vi "check running.vi"() -> ()   [LabVIEW 2025]
panel:
  out "running":u8
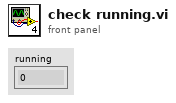
[diagram p1: front panel]
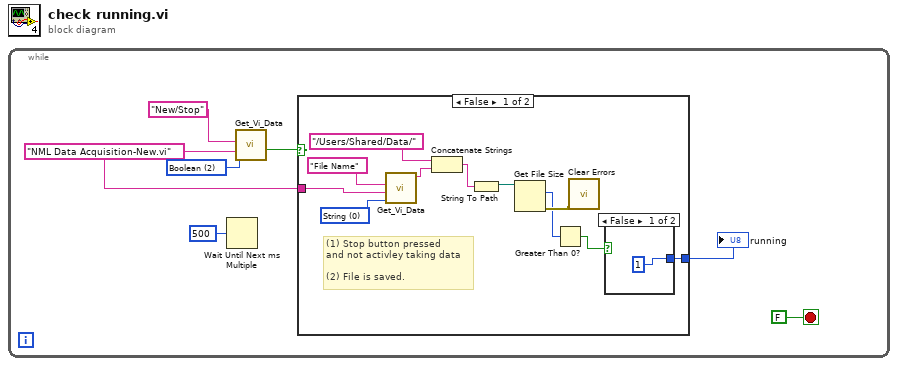
[diagram p0: block diagram]
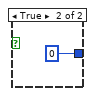
[diagram p2: hidden frame]
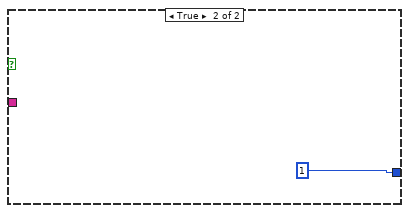
[diagram p3: hidden frame]
diagram:
  n1 = while {
    stop <- FALSE stop-if-true
    w6 = u16 2 items=["String", "Double", "Boolean", "Variant"] ("Data Type")
    w2 = "NML Data Acquisition-New.vi" ("VI name")
    n2 = Wait Until Next ms Multiple(millisecond multiple=u32 500) -> ()  [unwired: 1 out]
    n3 = call "Get_Vi_Data.vi"("Data Type"=w6, "VI name"=w2, "Control Name"="New/Stop") -> ("Boolean"=w5:bool)  [unwired: 4 in, 4 out]
    n4 = case shown="False" w5 {
      tunnel: w2 -> [w18 _]
      tunnel: [w12 u8 1 ("running")] -> w1
      frame False {
        w16 = u16 0 items=["String", "Double", "Boolean", "Variant"] ("Data Type")
        # "(1) Stop button pressed \nand not activley taking data\n\n(2) File is saved."
        n5 = call "Get_Vi_Data.vi"("Data Type"=w16, "VI name"=w18, "Control Name"="File Name") -> ("Data (String)"=w10:string)  [unwired: 4 in, 4 out]
        n6 = Concatenate Strings("/Users/Shared/Data/" ("string"), w10) -> (w9:string)
        n7 = String To Path(string=w9) -> (path=w15:path)
        n8 = Get File Size(file=w15) -> (size (in bytes)=w13:i64, 0:w14:errorcluster)  [unwired: 1 in, 1 out]
        n9 = Greater Than 0?(x=w13) -> (x > 0?=w11:bool)
        n10 = call <vilib>:"Clear Errors.vi"("error in (no error)"=w14) -> ()  [unwired: 5 in, 2 out]
        n11 = case shown="False" w11 {
          tunnel: [1 0] -> w12
          frame False {
          }
          frame True {
          }
        }
      }
      frame True {
      }
    }
    "running" <- w1
  }
